vi "Write GUI Events.vi"(8 "error in (no error)":errorcluster, 10 "GUI Events":T1, 11 "CS++DSMonitor in":refnum<class "CS++DSMonitor.lvclass">) -> (0 "error out":errorcluster, 3 "CS++DSMonitor out":refnum<class "CS++DSMonitor.lvclass">)   [LabVIEW 2015, in "CS++DSMonitor.lvlib" / "CS++DSMonitor.lvclass"]
doc: "Write GUI event references to attribute."
uses:
  CS++DSMonitor.lvclass
  <vilib>/ActorFramework/Message Enqueuer/Message Enqueuer.lvclass
  CS++PVMonitor Messages/CS++PVUpdate Msg/CS++PVUpdate Msg.lvclass
  CS++DSMonitor.lvclass/CS++DSMonitor.ctl
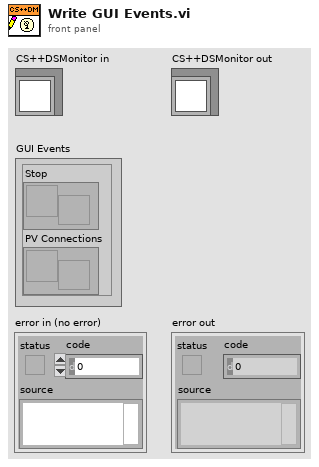
[diagram p1: front panel]
types:
  T1 = cluster{"Stop":refnum<user-event>, "PV Connections":refnum<user-event>}
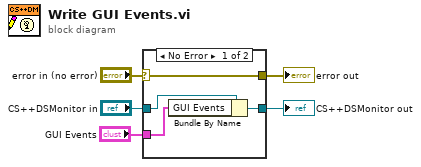
[diagram p0: block diagram]
diagram:
  n1 = case shown="No Error" "error in (no error)" {
    selector: "error in (no error)" -> [w9 w10]
    tunnel: [w9 w10] -> w4
    tunnel: [w7 w11] -> w2
    tunnel: "CS++DSMonitor in" -> [w8 w11]
    tunnel: "GUI Events" -> [w6 _]
    frame No Error {
      n2 = Bundle By Name(cluster=w8, "GUI Events"=w6) -> (w7:refnum<class "CS++DSMonitor.lvclass">)
    }
    frame Error {
    }
  }
  "error out" <- w4
  "CS++DSMonitor out" <- w2
